vi "Generate_REF_Waveforms.vi"(8 "error in (no error)":errorcluster, 9 "sampling info":cluster{"Fs":dbl, "#s":dbl}={"Fs"=1000.0, "#s"=1000.0} {"Fs" format="%.2p"}, 10 "reset signal":bool, 11 "lockin config":T1) -> (0 "error out":errorcluster, 3 "REF Waveforms":waveform(dbl)[](array[waveform]))   [LabVIEW 2016]
uses:
  Typedefs/lockin_config.ctl
  <vilib>/measure/NI_MABase.lvlib
  lockin.lvclass
panel:
  out "Numeric":i32
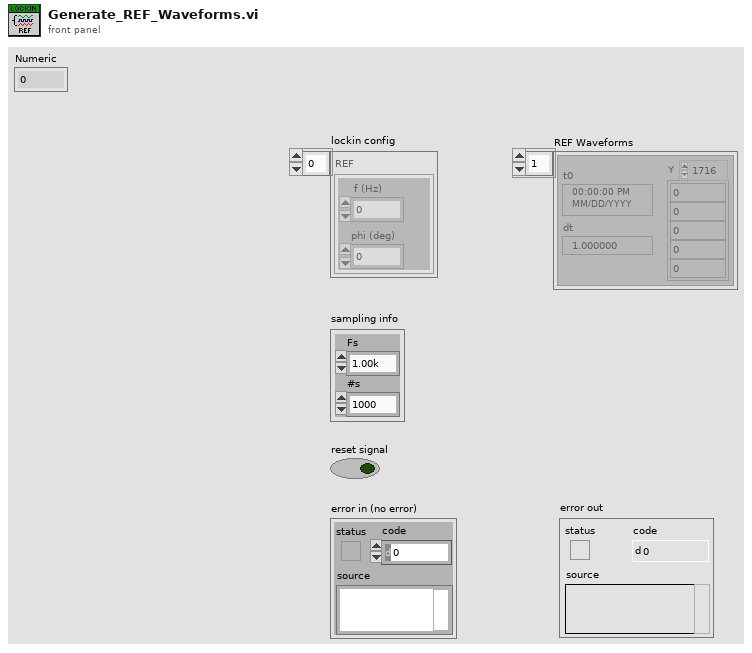
[diagram p1: front panel]
types:
  T1 = typedef "lockin.lvclass/lockin_config.ctl" = cluster{" f (Hz)":dbl, "phi (deg)":dbl}[]
  T2 = enum16{"Sine Wave", "Triangle Wave", "Square Wave", "Sawtooth Wave"}
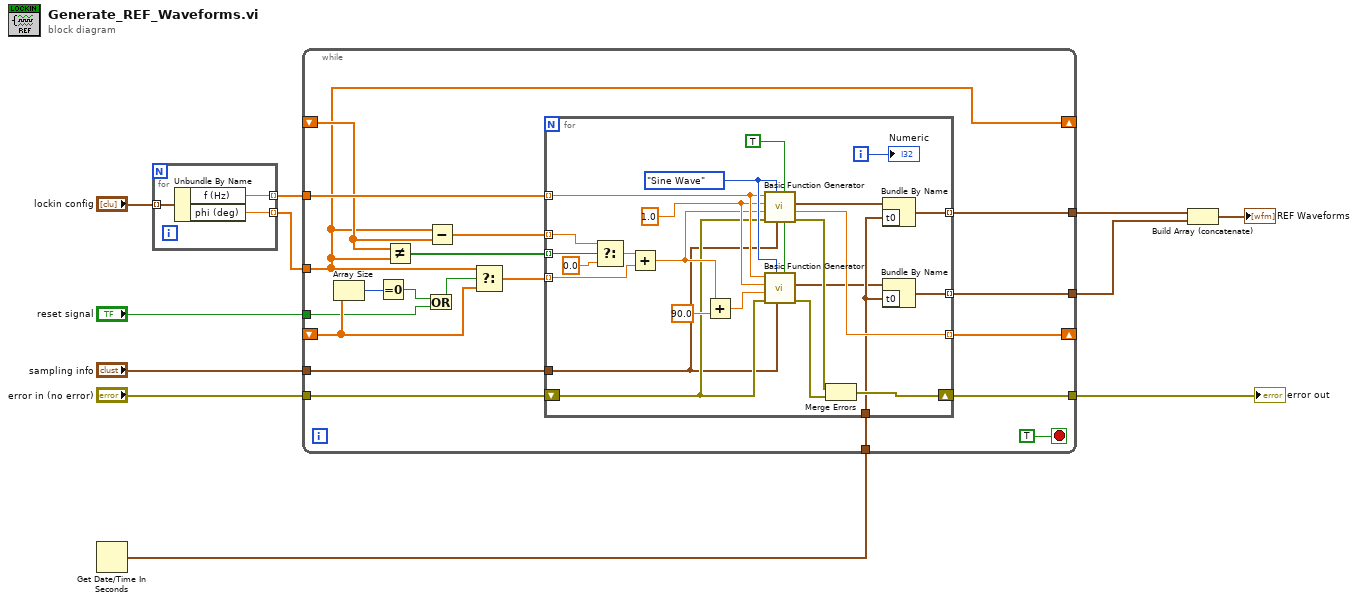
[diagram p0: block diagram]
diagram:
  n1 = Get Date/Time In Seconds() -> (seconds since 1Jan1904=w4:timestamp)
  n2 = for {
    tunnel: "lockin config" -> [w14] mode=indexing
    tunnel: [w13] -> w9 mode=indexing
    tunnel: [w12] -> w8 mode=indexing
    n3 = Unbundle By Name(w14) -> ("f (Hz)"=w13:dbl, "phi (deg)"=w12:dbl)
  }
  n4 = while {
    tunnel: "sampling info" -> [w18]
    tunnel: [w33] -> w3
    tunnel: w8 -> [w24]
    tunnel: w9 -> [w32]
    shift-right: [w24] -> _
    shift-left: _ -> [w29]
    shift-right: [w27] -> _
    shift-left: _ -> [w21]
    tunnel: w4 -> [w26]
    tunnel: "reset signal" -> [w19]
    tunnel: "error in (no error)" -> [w17]
    tunnel: [w16] -> w1
    tunnel: [w15] -> w2
    stop <- TRUE stop-if-true
    n5 = Array Size(array=w21) -> (size(s)=w25:i32)
    n6 = Equal To 0?(x=w25) -> (x = 0?=w20:bool)
    n7 = Not Equal?(x=w29, y=w24) -> (x != y?=w30:bool[])
    n8 = Or(x=w20, y=w19) -> (x .or. y?=w23:bool)
    n9 = Subtract(x=w24, y=w29) -> (x-y=w28:dbl[])
    n10 = Select(t=w24, s=w23, f=w21) -> (s? t:f=w22:dbl[])
    n11 = for {
      tunnel: w32 -> [w47] mode=indexing
      tunnel: [w51] -> w33 mode=indexing
      tunnel: w18 -> [w38]
      tunnel: w30 -> [w53] mode=indexing
      tunnel: w28 -> [w55] mode=indexing
      tunnel: [w50] -> w27 mode=indexing
      tunnel: w22 -> [w49] mode=indexing
      tunnel: w26 -> [w36]
      shift-right: [w37] -> w16
      shift-left: w17 -> [w41]
      tunnel: [w34] -> w15 mode=indexing
      i -> [w52]
      w48 = T2."Sine Wave" ("signal type")
      w45 = 1.0 ("amplitude")
      w46 = TRUE ("reset signal")
      n12 = Select(t=w55, s=w53, f=0.0) -> (s? t:f=w56:dbl)
      n13 = Add(x=w56, y=w49) -> (x+y=w44:dbl)
      n14 = Add(x=w44, y=90.0) -> (x+y=w42:dbl)
      n15 = call <vilib>:"Basic Function Generator.vi"("reset signal"=w46, "sampling info"=w38, "signal type"=w48, "error in (no error)"=w41, "phase"=w44, "amplitude"=w45, "frequency"=w47) -> ("error out"=w39:errorcluster, "phase out"=w50:dbl, "signal out"=w57:waveform(dbl))  [unwired: 2 in]
      n16 = call <vilib>:"Basic Function Generator.vi"("reset signal"=w46, "sampling info"=w38, "signal type"=w48, "error in (no error)"=w41, "phase"=w42, "amplitude"=w45, "frequency"=w47) -> ("error out"=w40:errorcluster, "signal out"=w35:waveform(dbl))  [unwired: 2 in, 1 out]
      n17 = Merge Errors(w39, w40) -> (w37:errorcluster)
      n18 = Bundle By Name(cluster=w57, "t0"=w36) -> (w51:waveform(dbl))
      n19 = Bundle By Name(cluster=w35, "t0"=w36) -> (w34:waveform(dbl))
      "Numeric" <- w52
    }
  }
  "error out" <- w1
  n20 = Build Array (concatenate)(w3, w2) -> (→"REF Waveforms":waveform(dbl)[])
